vi "grabber stage control panel.vi"() -> ()   [LabVIEW 2010]
uses:
  location3D.ctl
  ASI-stage/stage properties.ctl
panel:
  in  "large deviation override":T1={"x (um)"=600.0, "y (um)"=800.0, "Poverride"=1.2}
  out "file write error":bool
  out "file access error":bool
  out "error out":errorcluster
  in  "set pcros (um)":cluster{"X":dbl, "Y":dbl, "Z":dbl}={"X"=0.02, "Y"=0.02, "Z"=0.02}
  in  "deadband (um)":dbl=0.1
  out "tracker location":T2
  out "z move (um)":dbl
  out "y move (um)":dbl
  out "x move (um)":dbl
  in  "HALT":bool
  out "out of range":bool
  out "limits":T3
  out "stage initialized":bool
  in  "move stage":bool
  in  "target":cluster{"X ":dbl, "Y ":dbl, "Z ":dbl} {"Z" format="%#.4f"; "Y" format="%#.4f"; "X" format="%#.4f"}
  out "location":cluster{"X ":dbl, "Y ":dbl, "Z ":dbl} {"Z" format="%#.4f"; "Y" format="%#.4f"; "X" format="%#.4f"}
  in  "z range (um)":dbl=200.0
  in  "xy range (um)":dbl=10000.0
  in  "update period (ms)":u32=25
  in  "Baud rate":u32=115200
  in  "stage com port":refnum<visa-resource-name>="COM9"
  in  "set stage boundaries":bool
  in  "close stage":bool
  in  "open stage":bool
  in  "stop":bool
  out "stage location":cluster{"X out":dbl, "Y out":dbl, "Z out":dbl}(graph)
  in  "Z gains":T4={"proportional gain (Kc)"=0.35, "integral time (Ti, sec)"=15.0, "derivative time (Td, sec)"=0.0} {"derivative time (Td, sec)" format="%.3f"; "integral time (Ti, sec)" format="%.3f"; "proportional gain (Kc)" format="%.3f"}
  in  "XY gains":T4={"proportional gain (Kc)"=0.35, "integral time (Ti, sec)"=15.0, "derivative time (Td, sec)"=0.0} {"derivative time (Td, sec)" format="%.3f"; "integral time (Ti, sec)" format="%.3f"; "proportional gain (Kc)" format="%.3f"}
  in  "feedback polarity":T5={"x polarity"=TRUE, "y polarity"=FALSE, "z polarity"=FALSE}
  in  "engage stage feedback":bool
  out "tracking":bool
  in  "focalPositionQueue":refnum<queue>
  # "correct (tuned) parameters = 0.35, 15, 0"
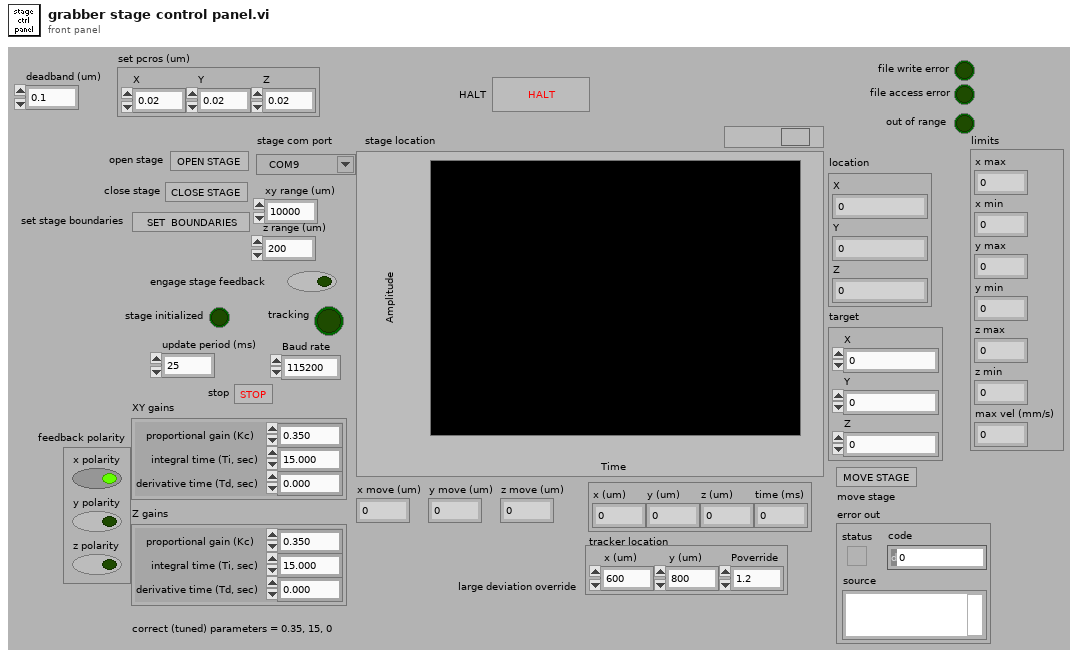
[diagram p1: front panel]
types:
  T1 = cluster{"x (um)":dbl, "y (um)":dbl, "Poverride":dbl}
  T2 = cluster{"x (um)":dbl, "y (um)":dbl, "z (um)":dbl, "time (ms)":i64}
  T3 = cluster{"x max":dbl, "x min":dbl, "y max":dbl, "y min":dbl, "z max":dbl, "z min":dbl, "max vel (mm/s)":dbl}
  T4 = cluster{"proportional gain (Kc)":dbl, "integral time (Ti, sec)":dbl, "derivative time (Td, sec)":dbl}
  T5 = cluster{"x polarity":bool, "y polarity":bool, "z polarity":bool}
  T6 = typedef "stage properties.ctl" = cluster{"VISA resource name":refnum<visa-resource-name>, "limits":cluster{"x max":dbl, "x min":dbl, "y max":dbl, "y min":dbl, "z max":dbl, "z min":dbl, "max vel (mm/s)":dbl}, "initialized":bool, "PCROS":cluster{"X":dbl, "Y":dbl, "Z":dbl}}
  T7 = typedef "location3D.ctl" = cluster{"x (um)":dbl, "y (um)":dbl, "z (um)":dbl, "time (ms)":i64}
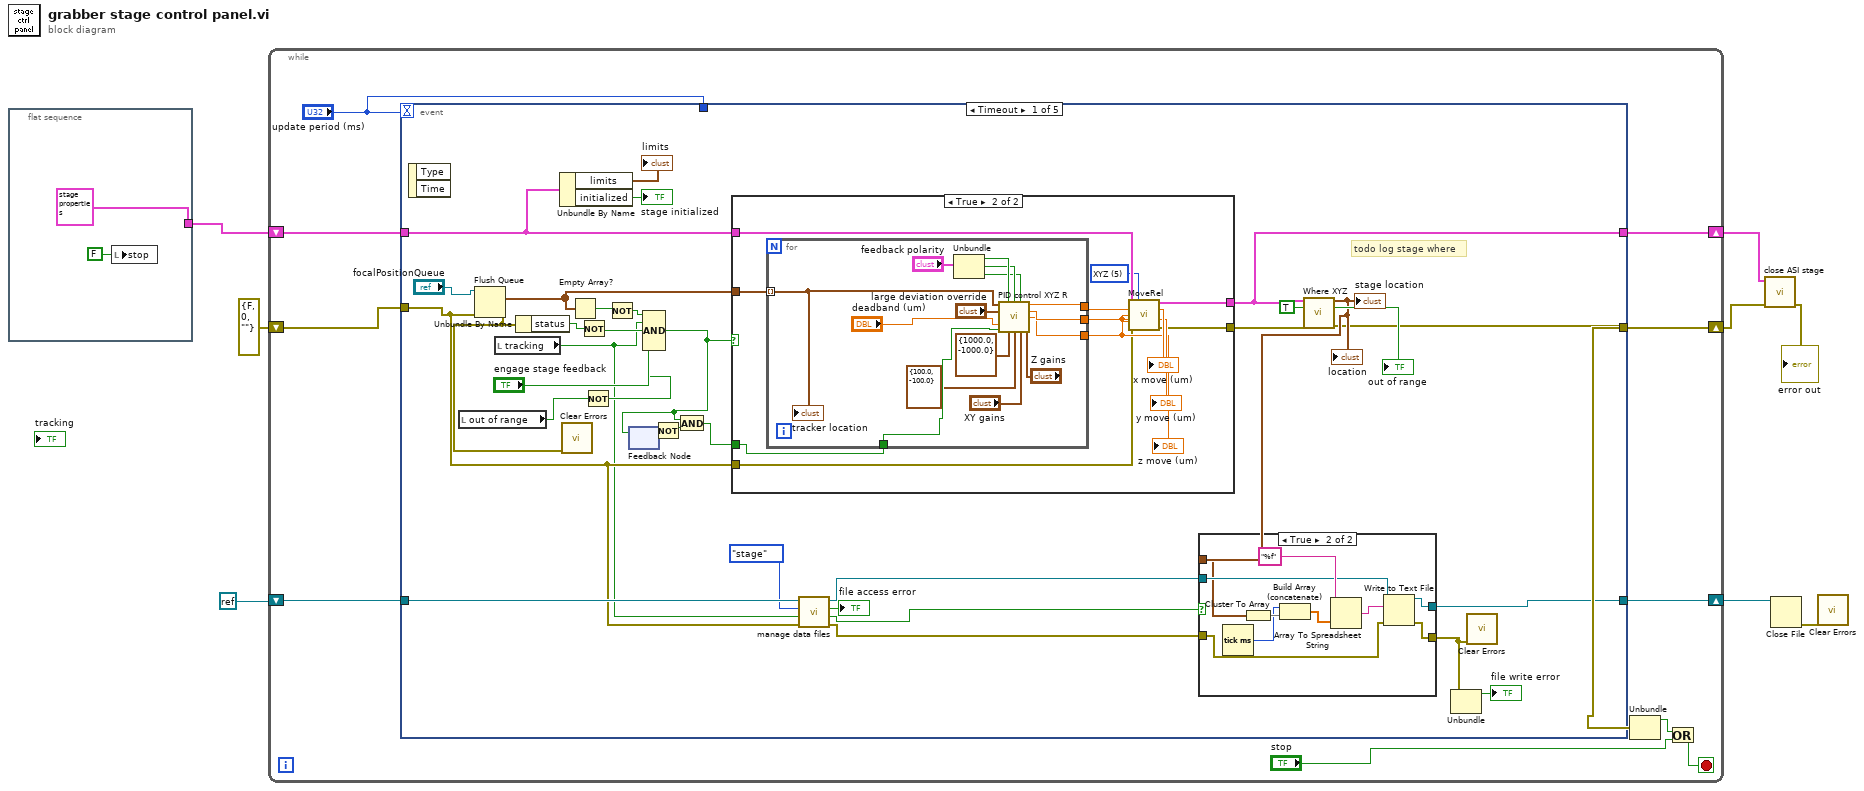
[diagram p0: block diagram]
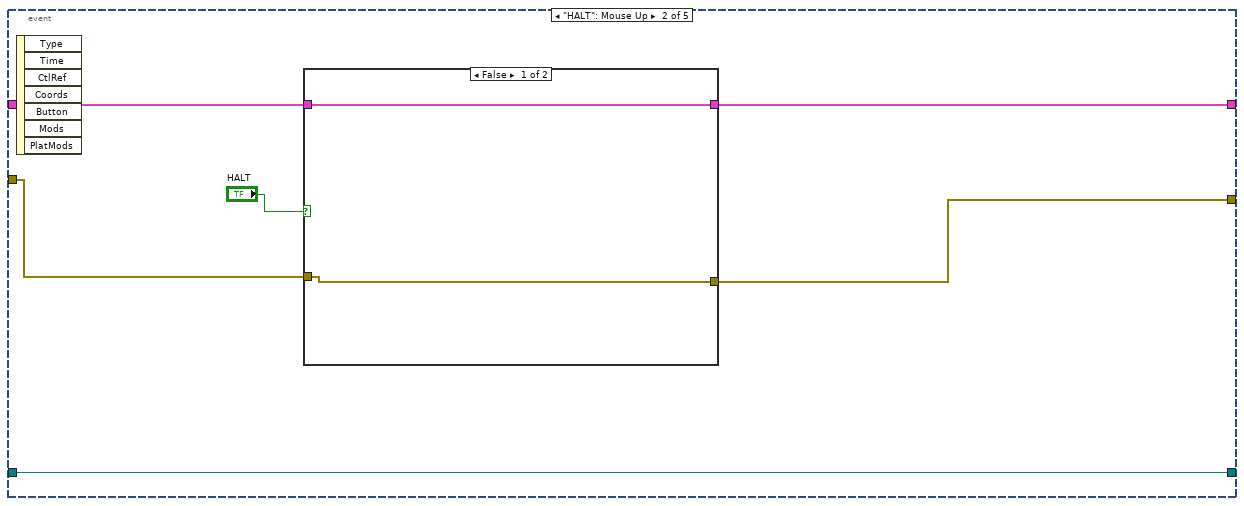
[diagram p4: hidden frame]
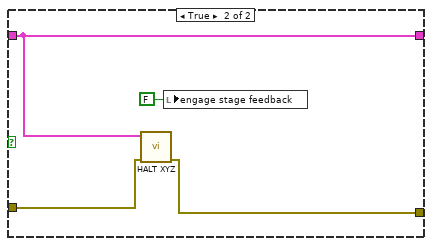
[diagram p5: hidden frame]
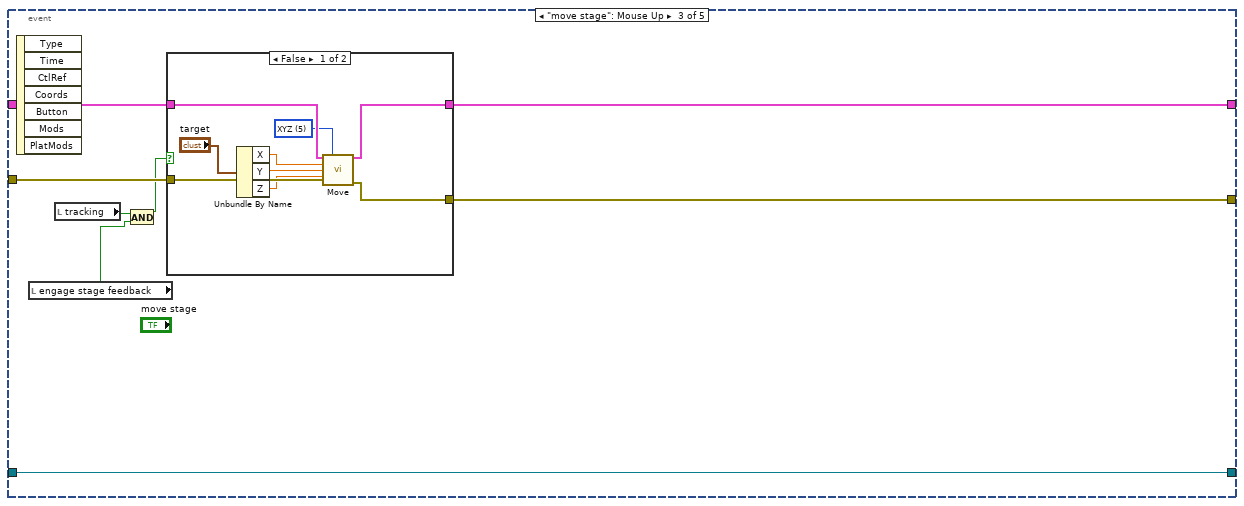
[diagram p6: hidden frame]
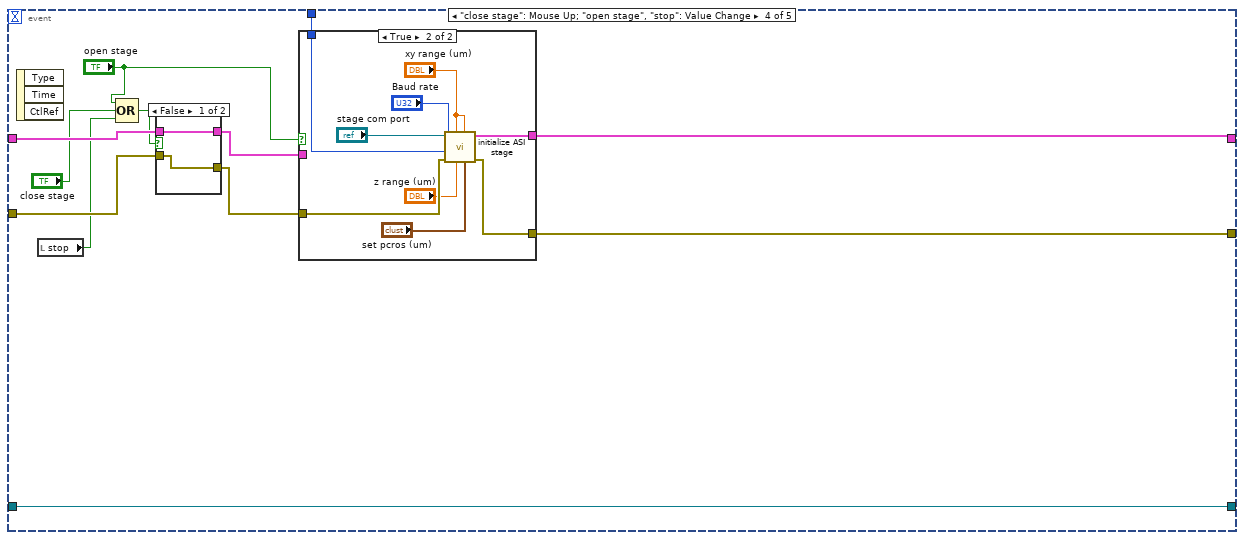
[diagram p8: hidden frame]
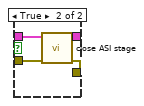
[diagram p9: hidden frame]
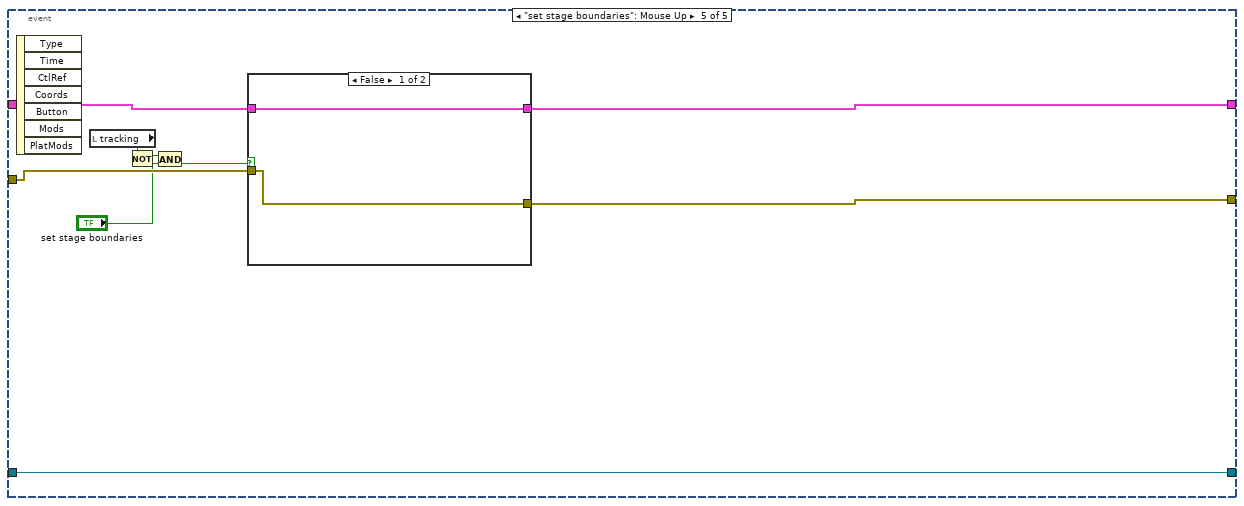
[diagram p11: hidden frame]
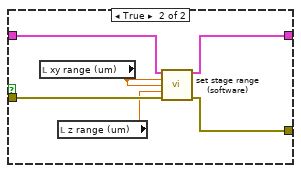
[diagram p12: hidden frame]
diagram:
  n1 = flat-sequence {
    tunnel: [T6 {"VISA resource name"="", "limits"={"x max"=0.0, "x min"=0.0, "y max"=0.0, "y min"=0.0, "z max"=0.0, "z min"=0.0, "max vel (mm/s)"=0.0}, "initialized"=FALSE, "PCROS"={"X"=0.0, "Y"=0.0, "Z"=0.0}} ("ASI stage")] -> w7
    frame #0 {
      n2 = local write "stop"(FALSE ("stop")) -> ()
    }
  }
  n3 = while {
    shift-right: [w17] -> w5
    shift-left: w7 -> [w19]
    shift-right: [w16] -> w6
    shift-left: errorcluster {"status"=FALSE, "code"=0, "source"=""} ("error out") -> [w18]
    shift-right: [w11] -> w2
    shift-left: refnum<k0> refnum -> [w10]
    stop <- w14 stop-if-true
    n4 = event shown="[0] Timeout" {
      selector: _ -> [_ _ _ _ _]
      dyn-events: _ -> [_ _ _ _ _]
      timeout: "update period (ms)" -> [_ _ _ _ _]
      tunnel: w19 -> [w43 w97 w111 w133 w161]
      tunnel: [w22 w95 w109 w135 w159] -> w16
      tunnel: w18 -> [w31 w96 w112 w132 w160]
      tunnel: [w44 w94 w110 w134 w158] -> w17
      tunnel: "update period (ms)" -> [_ _ _ w125 _]
      tunnel: [w23 w93 w105 w124 w153] -> w11
      tunnel: w10 -> [w32 w93 w105 w124 w153]
      event Timeout {
        # "todo log stage where"
        n5 = event-data() -> ()  [unwired: 1 in, 2 out]
        n6 = local read "out of range"() -> (w38:bool)
        n7 = Flush Queue(queue="focalPositionQueue", error in (no error)=w31) -> (remaining elements=w50:T7[], error out=w33:errorcluster)  [unwired: 1 out]
        n8 = local read "tracking"() -> (w29:bool)
        n9 = Unbundle By Name(w33) -> ("status"=w35:bool)
        n10 = Unbundle By Name(w43) -> ("limits"=→"limits":T3, "initialized"=→"stage initialized":bool)
        n11 = call <vilib>:"Clear Errors.vi"("error in (no error)"=w33) -> ()  [unwired: 6 in, 1 out]
        n12 = Empty Array?(array=w50) -> (empty?=w52:bool)
        n13 = Not(x=w35) -> (.not. x?=w34:bool)
        n14 = Not(x=w38) -> (.not. x?=w37:bool)
        n15 = Not(x=w52) -> (.not. x?=w51:bool)
        n16 = feedback #1() -> (w49:bool)  [unwired: 1 in]
        n17 = Compound Arithmetic op=AND(w51, w29, w34, "engage stage feedback", w37) -> (w36:bool)
        n18 = feedback-in #1(w36) -> ()
        n19 = Not(x=w49) -> (.not. x?=w48:bool)
        n20 = And(x=w36, y=w48) -> (x .and. y?=w47:bool)
        n21 = case shown="True" w36 {
          tunnel: w50 -> [_ w77]
          tunnel: w47 -> [_ w76]
          tunnel: w43 -> [w66 w75]
          tunnel: w31 -> [w67 w71]
          tunnel: [w67 w69] -> w46
          tunnel: [w66 w68] -> w44
          frame False {
          }
          frame True {
            w70 = u16 5 items=["No axis", "X", "Y", "Z", "XY", "XYZ"] ("Axis configuration")
            n22 = for {
              tunnel: w77 -> [w80] mode=indexing
              tunnel: w76 -> [w92]
              tunnel: [w83] -> w74
              tunnel: [w82] -> w73
              tunnel: [w81] -> w72
              n23 = Unbundle("feedback polarity") -> ("x polarity"=w90:bool, "y polarity"=w89:bool, "z polarity"=w88:bool)
              n24 = call "PID control XYZ R.vi"("location"=w80, "x polarity"=w90, "y polarity"=w89, "z polarity"=w88, "large deviation override"="large deviation override", "deadband (um)"="deadband (um)", "reinitialize? (F)"=w92, "XY pos range (um)"=cluster{"output high":dbl, "output low":dbl} {"output high"=1000.0, "output low"=-1000.0}, "z position range (um)"=cluster{"output high":dbl, "output low":dbl} {"output high"=100.0, "output low"=-100.0}, "XY gains"="XY gains", "Z gains"="Z gains") -> ("x move (um)"=w83:dbl, "y move (um)"=w82:dbl, "z move (um)"=w81:dbl)  [unwired: 2 in]
              "tracker location" <- w80
            }
            "x move (um)" <- w74
            "y move (um)" <- w73
            "z move (um)" <- w72
            n25 = call "MoveRel.vi"("ASI stage"=w75, "Axis configuration"=w70, "x"=w74, "y"=w73, "z"=w72, "error in (no error)"=w71) -> ("ASI stage out"=w68:T6, "error out"=w69:errorcluster)  [unwired: 8 in]
          }
        }
        n26 = call "manage data files.vi"("error in"=w31, "tracking"=w29, "recording type"=enum16{"tracking", "stage"}."stage", "refnum in"=w32) -> ("error out"=w26:errorcluster, "file open for writing"=w27:bool, "file access error"=→"file access error":bool, "refnum out"=w24:refnum<file>)  [unwired: 4 in]
        n27 = call "Where XYZ.vi"("ASI stage"=w44, "stop if out of range"=TRUE, "error in (no error)"=w46) -> ("location"=w25:cluster{"X out":dbl, "Y out":dbl, "Z out":dbl}, "out of range"=→"out of range":bool, "error out"=w22:errorcluster)  [unwired: 10 in]
        "stage location" <- w25
        "location" <- w25
        n28 = case shown="True" w27 {
          tunnel: w26 -> [w54 w61]
          tunnel: w25 -> [_ w59]
          tunnel: w24 -> [w55 w63]
          tunnel: [w55 w62] -> w23
          tunnel: [w54 w60] -> w21
          frame False {
          }
          frame True {
            n29 = Tick Count (ms)() -> (millisecond timer value=w57:u32)
            n30 = Cluster To Array(cluster=w59) -> (array=w58:dbl[])
            n31 = Build Array (concatenate)(w57, w58) -> (w56:dbl[])
            n32 = Array To Spreadsheet String(array=w56, 3:"%f" ("format (%.3f)")) -> (spreadsheet string=w64:string)  [unwired: 1 in]
            n33 = Write to Text File(file (use dialog)=w63, text=w64, error in=w61) -> (refnum out=w62:refnum<file>, error out=w60:errorcluster)  [unwired: 1 in, 1 out]
          }
        }
        n34 = Unbundle(w21) -> ("status"=→"file write error":bool)  [unwired: 2 out]
        n35 = call <vilib>:"Clear Errors.vi"("error in (no error)"=w21) -> ()  [unwired: 6 in, 1 out]
      }
      event "HALT": Mouse Up {
        n36 = event-data() -> ()  [unwired: 1 in, 7 out]
        n37 = case shown="False" "HALT" {
          tunnel: w97 -> [w100 w102]
          tunnel: w96 -> [w99 w104]
          tunnel: [w99 w103] -> w95
          tunnel: [w100 w102] -> w94
          frame False {
          }
          frame True {
            n38 = call "HALT XYZ.vi"("error in (no error)"=w104, "ASI stage"=w102) -> ("error out"=w103:errorcluster)  [unwired: 9 in]
            n39 = local write "engage stage feedback"(FALSE ("engage stage feedback")) -> ()
          }
        }
      }
      event "move stage": Mouse Up {
        n40 = event-data() -> ()  [unwired: 1 in, 7 out]
        n41 = local read "engage stage feedback"() -> (w106:bool)
        n42 = local read "tracking"() -> (w108:bool)
        n43 = And(x=w108, y=w106) -> (x .and. y?=w107:bool)
        n44 = case shown="False" w107 {
          tunnel: w112 -> [w121 w122]
          tunnel: w111 -> [w120 w123]
          tunnel: [w119 w123] -> w110
          tunnel: [w118 w122] -> w109
          frame False {
            w117 = u16 5 items=["No axis", "X", "Y", "Z", "XY", "XYZ"] ("Axis configuration")
            n45 = Unbundle By Name("target") -> ("X"=w115:dbl, "Y"=w114:dbl, "Z"=w113:dbl)
            n46 = call "Move.vi"("ASI stage"=w120, "Axis configuration"=w117, "x"=w115, "y"=w114, "z"=w113, "error in (no error)"=w121) -> ("ASI stage out"=w119:T6, "error out"=w118:errorcluster)  [unwired: 8 in]
          }
          frame True {
          }
        }
      }
      event "close stage": Mouse Up; "open stage", "stop": Value Change {
        n47 = event-data() -> ()  [unwired: 1 in, 3 out]
        n48 = local read "stop"() -> (w127:bool)
        n49 = Compound Arithmetic op=OR("open stage", "close stage", w127) -> (w126:bool)
        n50 = case shown="False" w126 {
          tunnel: w133 -> [w137 w141]
          tunnel: w132 -> [w136 w140]
          tunnel: [w136 w139] -> w131
          tunnel: [w137 w138] -> w130
          frame False {
          }
          frame True {
            n51 = call "close ASI stage.vi"("error in (no error)"=w140, "ASI stage"=w141) -> ("error out"=w139:errorcluster, "ASI stage out"=w138:T6)  [unwired: 8 in]
          }
        }
        n52 = case shown="True" "open stage" {
          tunnel: w131 -> [w142 w150]
          tunnel: [w142 w147] -> w135
          tunnel: [w143 w146] -> w134
          tunnel: w130 -> [w143 _]
          tunnel: w125 -> [_ w144]
          frame False {
          }
          frame True {
            n53 = call "initialize ASI stage.vi"("set pcros (um)"="set pcros (um)", "y range"="xy range (um)", "z range"="z range (um)", "x range"="xy range (um)", "error in (no error)"=w150, "timeout"=w144, "Baud rate"="Baud rate", "VISA resource name"="stage com port") -> ("error out"=w147:errorcluster, "ASI stage"=w146:T6)  [unwired: 2 in]
          }
        }
      }
      event "set stage boundaries": Mouse Up {
        n54 = event-data() -> ()  [unwired: 1 in, 7 out]
        n55 = local read "tracking"() -> (w157:bool)
        n56 = Not(x=w157) -> (.not. x?=w155:bool)
        n57 = And(x="set stage boundaries", y=w155) -> (x .and. y?=w156:bool)
        n58 = case shown="False" w156 {
          tunnel: w161 -> [w163 w169]
          tunnel: w160 -> [w162 w168]
          tunnel: [w162 w167] -> w159
          tunnel: [w163 w166] -> w158
          frame False {
          }
          frame True {
            n59 = local read "xy range (um)"() -> (w165:dbl)
            n60 = local read "z range (um)"() -> (w164:dbl)
            n61 = call "set stage range (software).vi"("ASI stage"=w169, "x range"=w165, "y range"=w165, "z range"=w164, "error in (no error)"=w168) -> ("ASI stage out"=w166:T6, "error out"=w167:errorcluster)  [unwired: 9 in]
          }
        }
      }
    }
    n62 = Unbundle(w16) -> ("status"=w15:bool)  [unwired: 2 out]
    n63 = Or(x=w15, y="stop") -> (x .or. y?=w14:bool)
  }
  "error out" <- w6
  n64 = call "close ASI stage.vi"("error in (no error)"=w6, "ASI stage"=w5) -> ()  [unwired: 8 in, 2 out]
  n65 = Close File(refnum=w2) -> (error out=w1:errorcluster)  [unwired: 1 in, 1 out]
  n66 = call <vilib>:"Clear Errors.vi"("error in (no error)"=w1) -> ()  [unwired: 6 in, 1 out]
